vi "test Parse EST Clusters into EST IP.vi"(8 "error in (no error)":errorcluster, 11 "TestCase in":refnum<class "Bitfile Parsing Test Case.lvclass">) -> (0 "error out":errorcluster, 3 "TestCase out":refnum<class "Bitfile Parsing Test Case.lvclass">)   [LabVIEW 2015, in "Bitfile Parsing Test Case.lvclass"]
uses:
  Bitfile Parsing Test Case.lvclass
  System Explorer/String Array Property.ctl
  <userlib>/_OpenG.lib/file/file.llb/Append Path to Root if Relative - Scalar__ogtk.vi
  <vilib>/addons/_JKI Toolkits/VI Tester/TestCase.llb/TestCase.lvclass
  System Explorer/Engine Simulation Toolkit System Explorer.lvlib
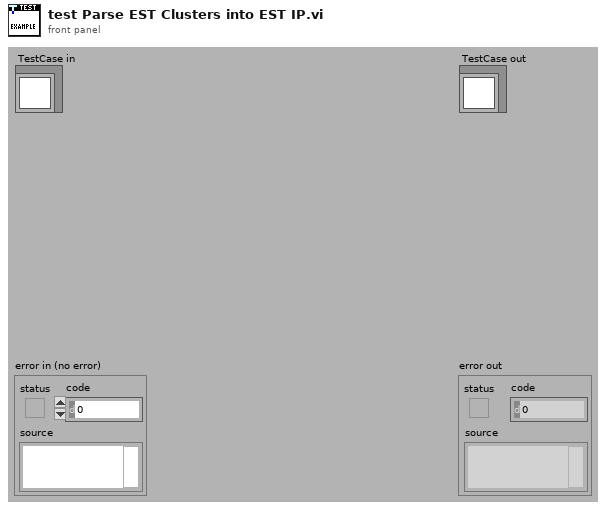
[diagram p1: front panel]
types:
  T1 = typedef "Engine Simulation Toolkit System Explorer.lvlib/String Array Property.ctl" = cluster{"Property Name":string, "Property Value":string[]}
  T2 = typedef "Engine Simulation Toolkit Shared.lvlib/Bitfile EST Version.ctl" = enum16{"1.0", "1.1", "1.2", "1.3", "1.4"}
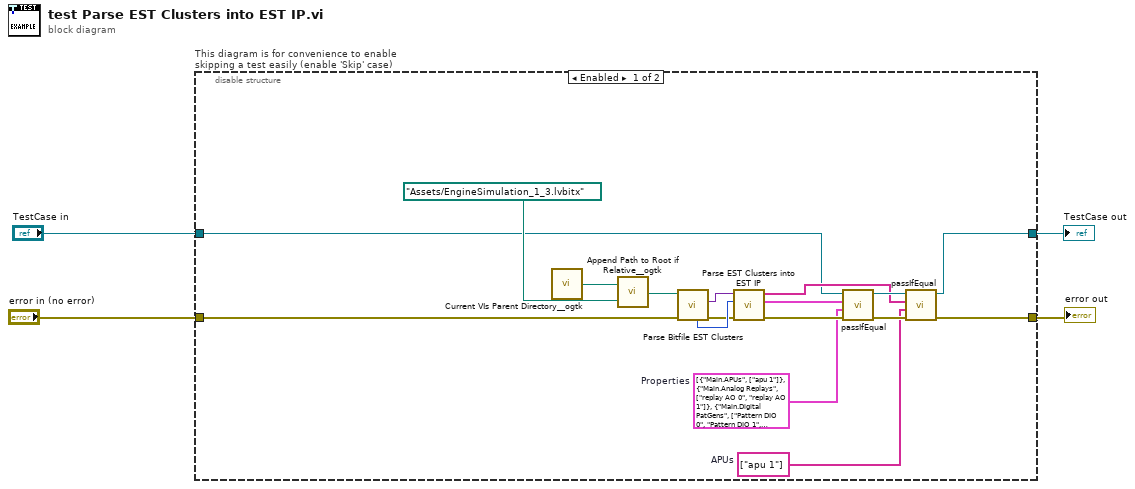
[diagram p0: block diagram]
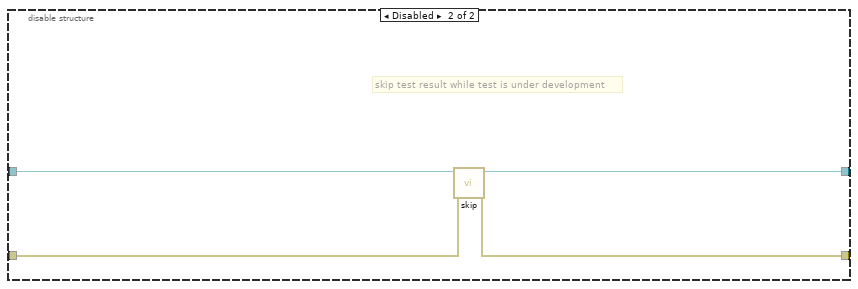
[diagram p2: hidden frame]
diagram:
  n1 = disable-structure "This diagram is for convenience to enable skipping a test easily (enable 'Skip' case)" shown="Enabled" {
    disable-tunnel: "TestCase in" -> [w6 w25]
    disable-tunnel: [w10 w23] -> w1
    disable-tunnel: [w12 w24] -> w3
    disable-tunnel: "error in (no error)" -> [w18 w22]
    frame Enabled {
      w5 = T1[] [{"Property Name"="Main.APUs", "Property Value"=["apu 1"]}, {"Property Name"="Main.Analog Replays", "Property Value"=["replay AO 0", "replay AO 1"]}, {"Property Name"="Main.Digital PatGens", "Property Value"=["Pattern DIO 0", "Pattern DIO 1", "Pattern DIO 2", "Pattern DIO 3"]}, {"Property Name"="Main.ETiming Caps", "Property Value"=["Event DIO 4.Event 1", "Event DIO 5.Event 1", "Event DIO 6.Event 1", "Event DIO 7.Event 1", "Event DIO 8.Event 1", "Event DIO 9.Event 1", "Multi Event DIO 10.Event 1", "Multi Event DIO 10.Event 2", "Multi Event DIO 10.Event 3", "Multi Event DIO 10.Event 4", "Multi Event DIO 11.Event 1", "Multi Event DIO 11.Event 2", "Multi Event DIO 11.Event 3", "Multi Event DIO 11.Event 4", "Multi Event DIO 12.Event 1", "Multi Event DIO 12.Event 2", "Multi Event DIO 12.Event 3", "Multi Event DIO 12.Event 4", "Multi Event DIO 13.Event 1", "Multi Event DIO 13.Event 2", "Multi Event DIO 13.Event 3", "Multi Event DIO 13.Event 4", "Multi Event DIO 14.Event 1", "Multi Event DIO 14.Event 2", "Multi Event DIO 14.Event 3", "Multi Event DIO 14.Event 4", "Multi Event DIO 15.Event 1", "Multi Event DIO 15.Event 2", "Multi Event DIO 15.Event 3", "Multi Event DIO 15.Event 4"]}, {"Property Name"="Main.ETiming Meas", "Property Value"=["Event DIO 4", "Event DIO 5", "Event DIO 6", "Event DIO 7", "Event DIO 8", "Event DIO 9", "Multi Event DIO 10", "Multi Event DIO 11", "Multi Event DIO 12", "Multi Event DIO 13", "Multi Event DIO 14", "Multi Event DIO 15"]}, {"Property Name"="Main.Knock Cylinder", "Property Value"=["Knock AO 2.Cylinder 1", "Knock AO 2.Cylinder 2", "Knock AO 2.Cylinder 3", "Knock AO 2.Cylinder 4", "Knock AO 2.Cylinder 5", "Knock AO 2.Cylinder 6", "Knock AO 3.Cylinder 1", "Knock AO 3.Cylinder 2", "Knock AO 3.Cylinder 3", "Knock AO 3.Cylinder 4", "Knock AO 3.Cylinder 5", "Knock AO 3.Cylinder 6"]}, {"Property Name"="Main.Knock Sensor", "Property Value"=["Knock AO 2", "Knock AO 3"]}, {"Property Name"="Main.DirSpeed Sensor", "Property Value"=["Dir Speed DIO0", "Dir Speed DIO1"]}]  # Properties
      w8 = string[] ["apu 1"]  # APUs
      n2 = call <userlib>:"Current VIs Parent Directory__ogtk.vi"() -> ("Parent Directory (+ Relative)"=w21:path)  [unwired: 5 in]
      n3 = call-poly <userlib>:"Append Path to Root if Relative__ogtk.vi"("Absolute or Relative Path"=path "Assets/EngineSimulation_1_3.lvbitx" ("bitfile path"), "Root Path"=w21) -> ("Absolute or Appended Path"=w19:path)
      n4 = call "Parse Bitfile EST Clusters.vi"("error in (no error)"=w18, "bitfile path"=w19) -> ("error out"=w15:errorcluster, "EPS IP LUT"=w17:variant, "EST version enum"=w16:T2)  [unwired: 5 in, 2 out]
      n5 = call "Parse EST Clusters into EST IP.vi"("error in (no error)"=w15, "EST version enum"=w16, "EPS IP LUT"=w17) -> ("error out"=w7:errorcluster, "Properties"=w14:T1[], "APUs"=w9:string[])  [unwired: 6 in]
      n6 = call-dynamic "passIfEqual.vi"("error in (no error)"=w7, "y"=w5, "x"=w14, "TestCase in"=w6) -> ("error out"=w13:errorcluster, "TestCase out"=w11:refnum<class "Bitfile Parsing Test Case.lvclass">)  [unwired: 6 in]
      n7 = call-dynamic "passIfEqual.vi"("error in (no error)"=w13, "y"=w8, "x"=w9, "TestCase in"=w11) -> ("error out"=w12:errorcluster, "TestCase out"=w10:refnum<class "Bitfile Parsing Test Case.lvclass">)  [unwired: 6 in]
    }
    frame Disabled {
      # "skip test result while test is under development"
      n8 = call <vilib>:"skip.vi"("error in (no error)"=w22, "TestCase in"=w25) -> ("error out"=w24:errorcluster, "TestCase out"=w23:refnum<class "Bitfile Parsing Test Case.lvclass">)  [unwired: 8 in]
    }
  }
  "error out" <- w3
  "TestCase out" <- w1
